vi "get freq ring.vi"(8 "error in (no error)":errorcluster caption="에러 입력(에러 없음)", 11 "DW7802 입력":refnum<class "DW7802.lvclass">) -> (0 "error out":errorcluster caption="에러 출력", 1 "caption":string="PWM", 2 "strings & values":T1=[{"String"="12kHz", "Value"=12000}, {"String"="24kHz", "Value"=24000}, {"String"="48kHz", "Value"=48000}], 3 "DW7802 출력":refnum<class "DW7802.lvclass">, 4 "read value":u32=48000)   [LabVIEW 2020, in "DW7802.lvclass"]
uses:
  DW7802.lvclass
  <vilib>/Utility/miscctls.llb/LVStringsAndValuesArrayTypeDef_U32.ctl
  Haptic IC/Haptic IC.lvclass/Haptic IC.ctl
  SubVIs/I2C/Instance VIs/(SubVI)I2C_8Bit-8Bit_Read_Single.vi
  Haptic IC/Haptic IC.lvclass
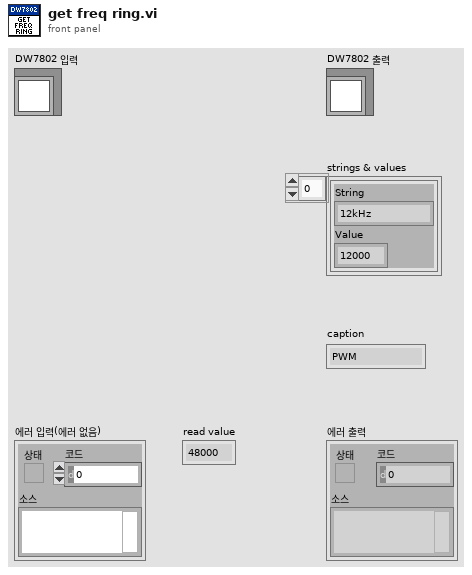
[diagram p1: front panel]
types:
  T1 = typedef "LVStringsAndValuesArrayTypeDef_U32.ctl" = cluster{"String":string, "Value":u32}[]
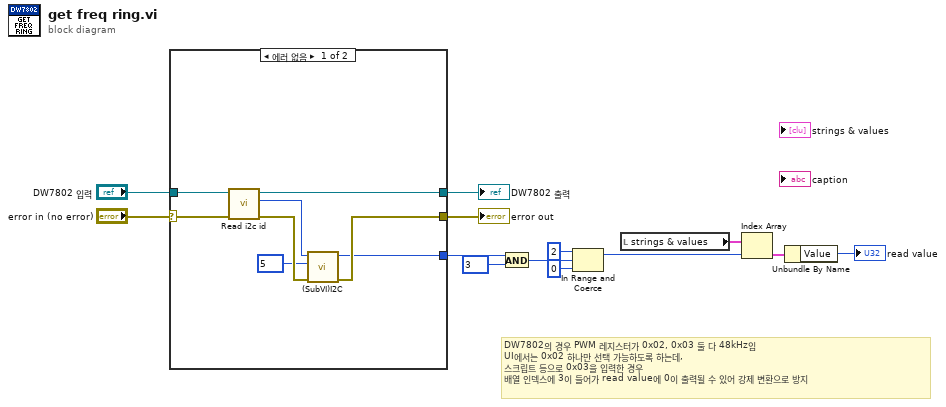
[diagram p0: block diagram]
diagram:
  # "DW7802의 경우 PWM 레지스터가 0x02, 0x03 둘 다 48kHz임\nUI에서는 0x02 하나만 선택 가능하도록 하는데, \n스크립트 등으로 0x03을 입력한 경우\n배열 인덱스에 3이 들어가 read value에 0이 출력될 수 있어 강제 변환으로 방지"
  n1 = case shown="에러 없음" "error in (no error)" {
    selector: "error in (no error)" -> [w20 w22]
    tunnel: "DW7802 입력" -> [w21 w23]
    tunnel: [w19 w23] -> w12
    tunnel: [w15 w22] -> w13
    tunnel: [w14 _] -> w7
    frame No Error {
      n2 = call "Read i2c id.vi"("error in (no error)"=w20, "Haptic IC 입력"=w21) -> ("error out"=w18:errorcluster, "i2c id"=w17:u8, "Haptic IC 출력"=w19:refnum<class "DW7802.lvclass">)  [unwired: 7 in]
      n3 = call-poly "(SubVI)I2C.vi"("error in (no error)"=w18, "Address"=u8 5, "ID"=w17) -> ("error out"=w15:errorcluster, "Read Data"=w14:u8)  [unwired: 6 in, 1 out]
    }
    frame Error {
    }
  }
  "error out" <- w13
  "DW7802 출력" <- w12
  n4 = And(x=w7, y=u8 3) -> (x .and. y?=w8:u8)
  n5 = In Range and Coerce(upper limit=u8 2 ("상위 리미트"), x=w8, lower limit=u8 0 ("하위 리미트")) -> (coerced(x)=w3:u8)  [unwired: 1 out]
  n6 = local read "strings & values"() -> (w6:T1)
  n7 = Index Array(array=w6, index=w3) -> (element=w5:cluster{"String":string, "Value":u32})
  n8 = Unbundle By Name(w5) -> ("Value"=→"read value":u32)
